vi "Log Data I8.vi"(0 "TDMS Log In":refnum<class "TDMS Logger.lvclass">, 5 "Group Name":string, 7 "Channels Names":string[](array[string]), 9 "I8 Data":i8[][](array[numeric]), 11 "Error In":errorcluster) -> (4 "TDMS Log Out":refnum<class "TDMS Logger.lvclass">, 15 "Error Out":errorcluster)   [LabVIEW 2019, in "TDMS Logger.lvlib" / "TDMS Logger.lvclass"]
doc: "Send I8 data to asynch logger."
uses:
  TDMS Logger.lvclass
  TDMS Logger.lvclass/TDMS Logger.ctl
  _Typedefs/Log Message.ctl
  _Typedefs/Log Action.ctl
  _Typedefs/Data Type.ctl
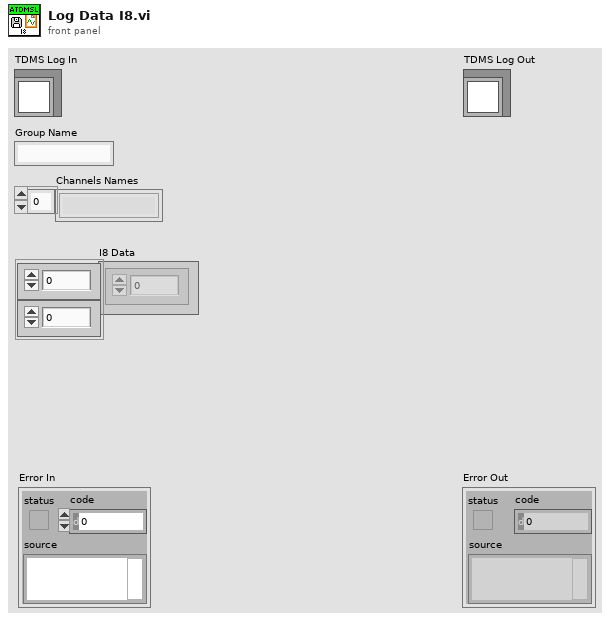
[diagram p1: front panel]
types:
  T1 = typedef "TDMS Logger.lvlib/TDMS Logger.lvclass/Data Type.ctl" = enum16{"I16", "I8", "String", "U16", "U8", "Waveform", "Double", "Single"}
  T2 = typedef "TDMS Logger.lvlib/TDMS Logger.lvclass/Log Action.ctl" = enum16{"Handle Old Files", "Status Update", "Stop", "Log Data", "Initialize"}
  T3 = typedef "TDMS Logger.lvlib/TDMS Logger.lvclass/Log Message.ctl" = cluster{"Log Action":T2, "Variant":variant, "Data Type":T1, "Group Name":string, "Channels Names":string[]}
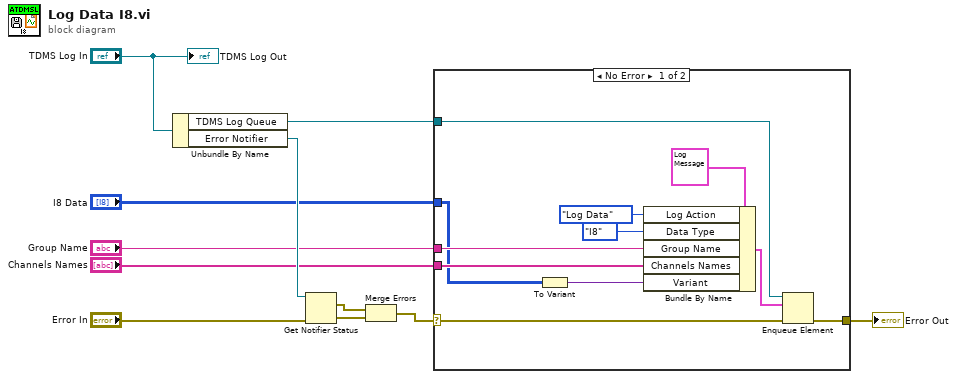
[diagram p0: block diagram]
diagram:
  n1 = Unbundle By Name("TDMS Log In") -> ("TDMS Log Queue"=w10:refnum<queue>, "Error Notifier"=w7:refnum<notifier>)
  n2 = Get Notifier Status(notifier=w7, error in (no error)="Error In") -> (current notification=w4:errorcluster, error out=w5:errorcluster)  [unwired: 3 out]
  n3 = Merge Errors(w4, w5) -> (w6:errorcluster)
  n4 = case shown="No Error" w6 {
    selector: w6 -> [w14 w23]
    tunnel: [w20 w23] -> w11
    tunnel: w10 -> [w19 _]
    tunnel: "I8 Data" -> [w13 _]
    tunnel: "Group Name" -> [w16 _]
    tunnel: "Channels Names" -> [w15 _]
    frame No Error {
      n5 = To Variant(anything=w13) -> (Variant=w12:variant)
      n6 = Bundle By Name(cluster=T3 {"Log Action"=enum."Stop", "Variant"=variant, "Data Type"=enum."String", "Group Name"="", "Channels Names"=[]} ("element"), "Log Action"=Log_Action."Log Data", "Data Type"=Data_Type."I8", "Group Name"=w16, "Channels Names"=w15, "Variant"=w12) -> (w21:T3)
      n7 = Enqueue Element(queue=w19, element=w21, error in (no error)=w14) -> (error out=w20:errorcluster)  [unwired: 1 in, 2 out]
    }
    frame Error {
    }
  }
  "Error Out" <- w11
  "TDMS Log Out" <- "TDMS Log In"
